vi "Create And Register Generic Method Server Event.vi"(8 "error in (no error)":errorcluster, 11 "gRPCid server in":T1) -> (0 "error out":errorcluster, 2 "Generic Method Event":refnum<user-event>, 3 "gRPCid server out":T1)   [LabVIEW 2019, in "Template Client.lvlib" / "gprc-lvsupport.lvlib"]
uses:
  gprc-lvsupport.lvlib
  typeDefs/grpcId.ctl
  typeDefs/Generic Method Event Data.ctl
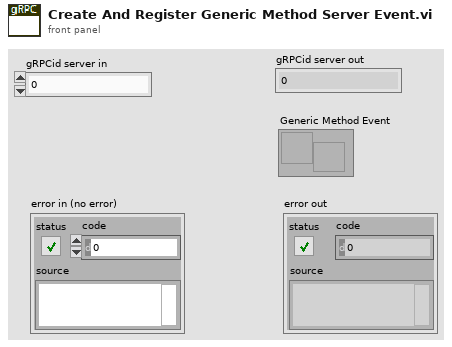
[diagram p1: front panel]
types:
  T1 = typedef "Template Client.lvlib/gprc-lvsupport.lvlib/grpcId.ctl" = u64
  T2 = typedef "Template Client.lvlib/gprc-lvsupport.lvlib/Generic Method Event Data.ctl" = cluster{"Method Name":string, "Method gRPCid":T1}
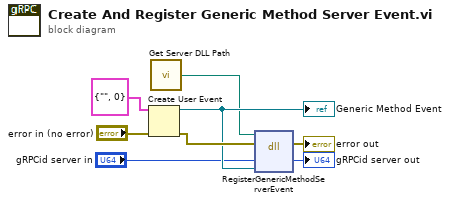
[diagram p0: block diagram]
diagram:
  n1 = Create User Event(user event datatype=T2 {"Method Name"="", "Method gRPCid"=0} ("Generic Method Event Data"), error in="error in (no error)") -> (user event=w6:refnum<user-event>, error out=w7:errorcluster)
  "Generic Method Event" <- w6
  n2 = call "Get Server DLL Path.vi"() -> ("Server dll path"=w2:path)
  n3 = dll-call lib="?" fn="RegisterGenericMethodServerEvent"(path in=w2, error in=w7, "serverId"="gRPCid server in", "genericMethodEvent"=w6) -> (error out=→"error out":errorcluster, "serverId"=→"gRPCid server out":T1)  [unwired: 3 in, 1 out]
